vi "Lockin.DAQ.Trigger.vi"(8 "error in (no error)":errorcluster, 11 "Lockin.DAQ":refnum<class "Lockin.DAQ.lvclass">) -> (0 "error out":errorcluster, 3 "Lockin.DAQ":refnum<class "Lockin.DAQ.lvclass">)   [LabVIEW 2016, in "Lockin.DAQ.lvclass"]
uses:
  Lockin.DAQ.lvclass
  Typedefs/DAQType-enum.ctl
  Lockin.DAQ.lvclass/Lockin.DAQ.ctl
  <vilib>/DAQmx/configure/trigger.llb/DAQmx Start Trigger (Digital Edge).vi
  <userlib>/_OpenG.lib/array/array.llb/Remove Duplicates from 1D Array (Variant)__ogtk.vi
  <resource>/objmgr/daqmx.rc
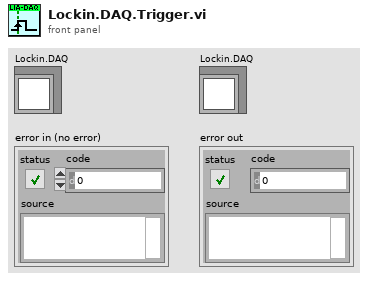
[diagram p1: front panel]
types:
  T1 = typedef "Lockin.DAQ.lvclass/DAQType-enum.ctl" = enum16{"None", "USB 4431", "PXI 446x"}
  T2 = cluster{"DAQ Type":T1, "Master Tasks":refnum<k21>[], "RefClk.Src":tag, "SyncPulse.Src":tag, "Trigger.Src":tag, "SyncPulse.SyncTime":dbl}
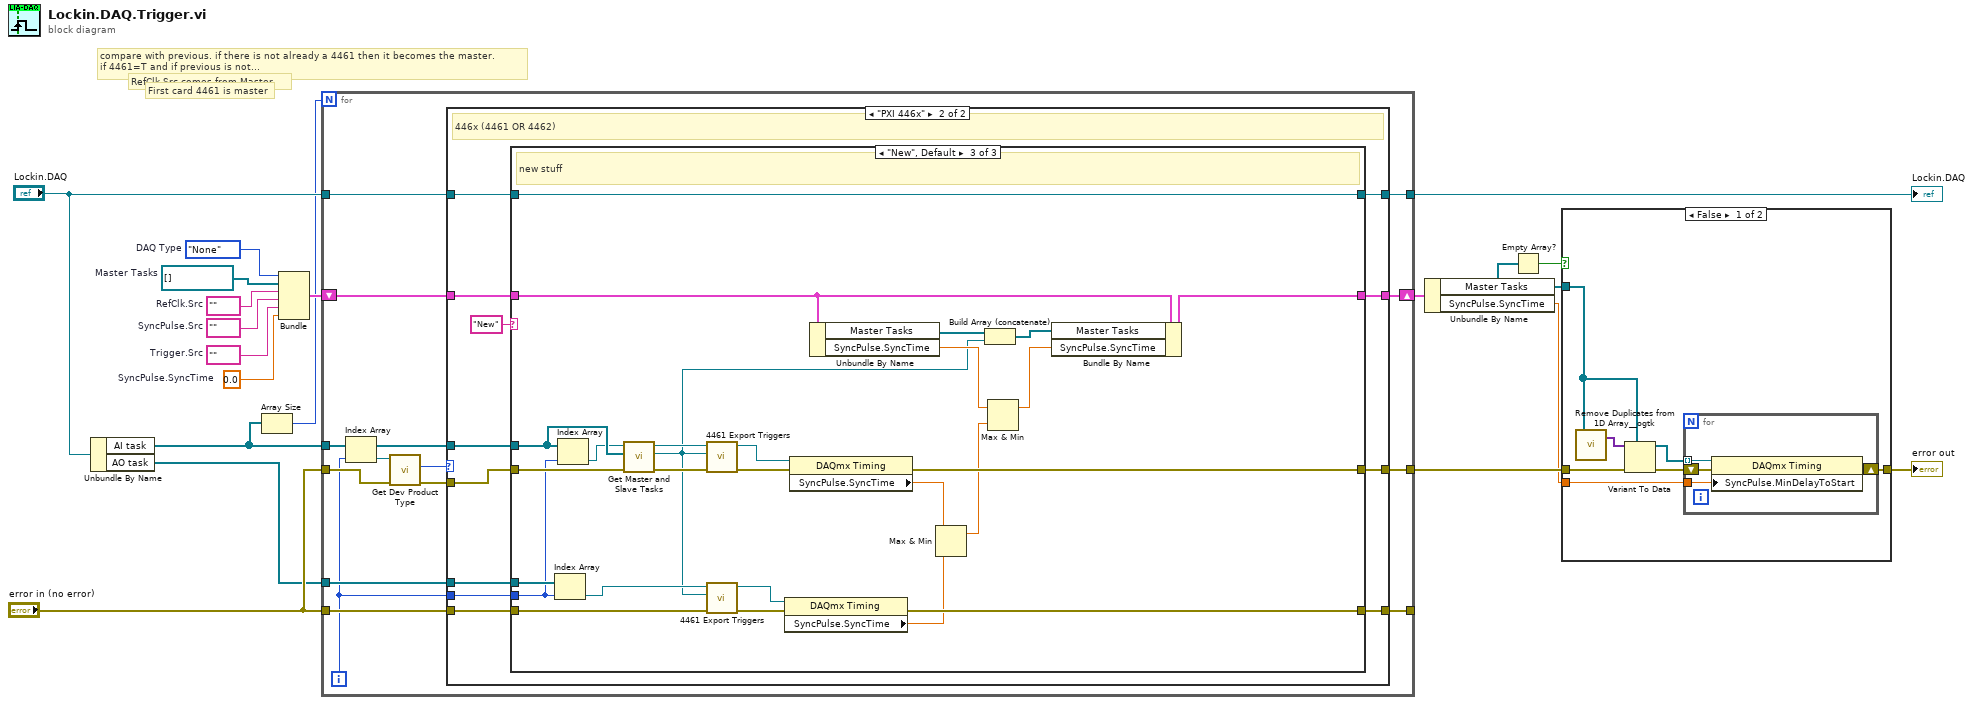
[diagram p0: block diagram]
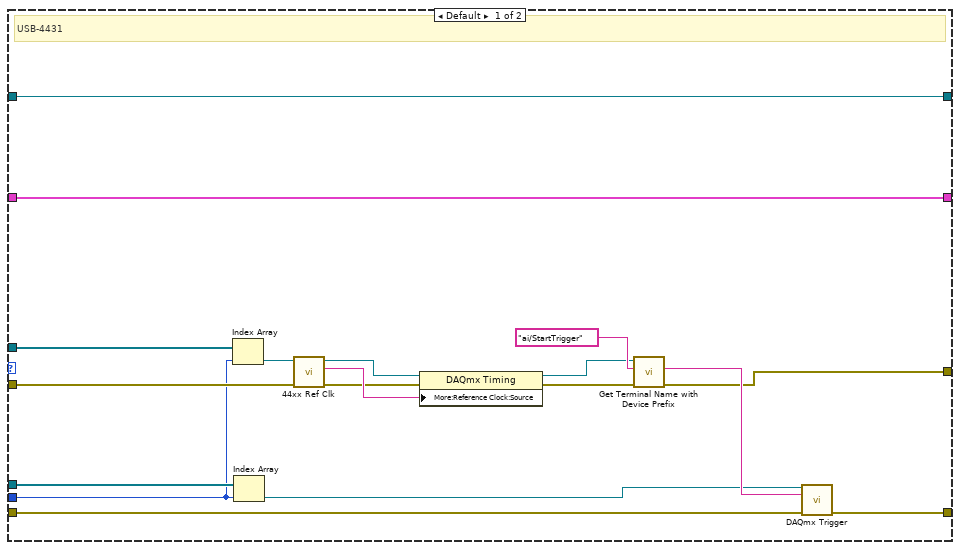
[diagram p2: hidden frame]
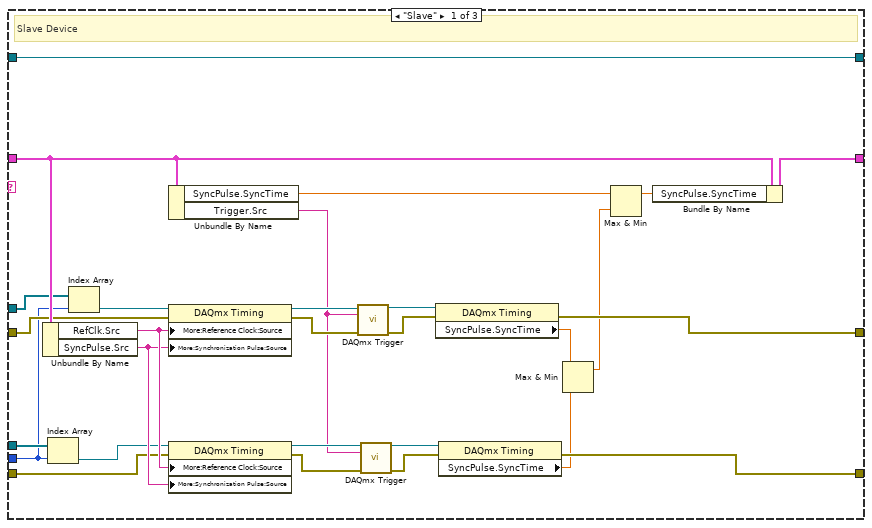
[diagram p3: hidden frame]
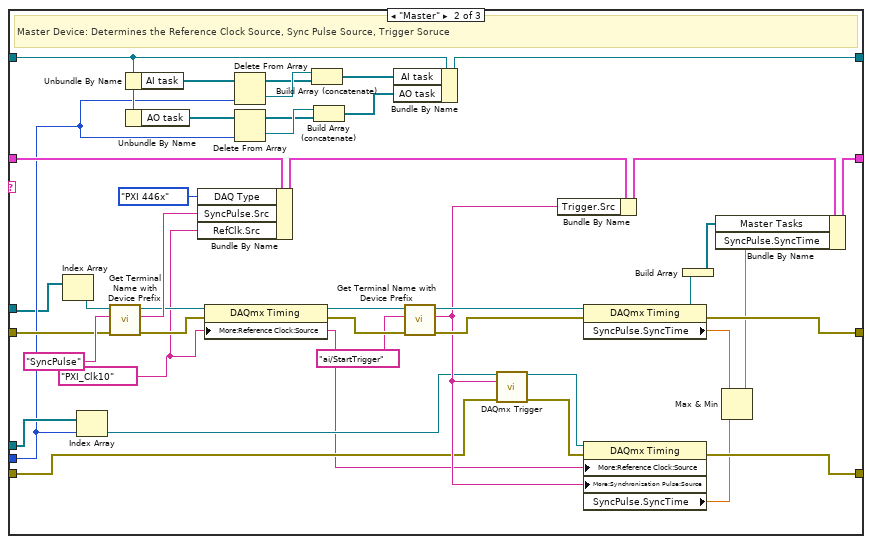
[diagram p4: hidden frame]
diagram:
  w1 = refnum<k21>[] []  # Master Tasks
  w13 = 0.0  # SyncPulse.SyncTime
  w12 = tag ""  # Trigger.Src
  w11 = tag ""  # SyncPulse.Src
  w5 = tag ""  # RefClk.Src
  w4 = DAQType-enum."None"  # DAQ Type
  # "RefClk.Src comes from Master"
  # "compare with previous. if there is not already a 4461 then it becomes the master. \nif 4461=T and if previous is not..."
  # "First card 4461 is master"
  n1 = Unbundle By Name("Lockin.DAQ") -> ("AI task"=w2:refnum<k21>[], "AO task"=w6:refnum<k21>[])
  n2 = Array Size(array=w2) -> (size(s)=w3:i32)
  n3 = Bundle("DAQ Type"=w4, "Master Tasks"=w1, "RefClk.Src"=w5, "SyncPulse.Src"=w11, "Trigger.Src"=w12, "SyncPulse.SyncTime"=w13) -> (w10:T2)  [unwired: 1 in]
  n4 = for {
    N: w3 -> [_]
    tunnel: w2 -> [w21]
    tunnel: "error in (no error)" -> [w33]
    shift-right: [w31] -> w14
    shift-left: w10 -> [w32]
    tunnel: [w30] -> w18
    tunnel: "Lockin.DAQ" -> [w29]
    tunnel: [w28] -> w8
    tunnel: [w27] -> _
    tunnel: "error in (no error)" -> [w26]
    tunnel: w6 -> [w23]
    i -> [w22]
    n5 = Index Array(array=w21, index=w22) -> (element=w24:refnum<k21>)
    n6 = call "Get Dev Product Type.vi"("error in (no error)"=w33, "Refnum in"=w24) -> ("error out"=w20:errorcluster, "DAQ Type"=w25:T1)  [unwired: 6 in, 2 out]
    n7 = case shown="\"PXI 446x\"" w25 {
      tunnel: w32 -> [w51 w63]
      tunnel: [w51 w62] -> w31
      tunnel: w20 -> [w38 w61]
      tunnel: [w42 w60] -> w30
      tunnel: w29 -> [w50 w59]
      tunnel: [w50 w58] -> w28
      tunnel: [w43 w55] -> w27
      tunnel: w26 -> [w44 w57]
      tunnel: w23 -> [w46 w56]
      tunnel: w22 -> [w35 w54]
      tunnel: w21 -> [w36 w53]
      frame Default {
        # "USB-4431"
        n8 = Index Array(array=w36, index=w35) -> (element=w34:refnum<k21>)
        n9 = Index Array(array=w46, index=w35) -> (element=w41:refnum<k21>)
        n10 = call "44xx Ref Clk.vi"("error in (no error)"=w38, "Refnum in"=w34) -> ("error out"=w37:errorcluster, "RefClk.Src"=w40:tag, "Refnum out"=w39:refnum<k21>)  [unwired: 7 in]
        n11 = property class="DAQmx Timing"(reference=w39, error in=w37, "More:Reference Clock:Source"=w40) -> (reference out=w48:refnum<k21>, error out=w47:errorcluster)
        n12 = call "Get Terminal Name with Device Prefix.vi"("error in (no error)"=w47, "Local Terminal Name"="ai/StartTrigger", "task/channels in"=w48) -> ("error out"=w42:errorcluster, "Terminal Name with Device Prefix"=w45:tag)  [unwired: 6 in, 1 out]
        n13 = call-poly <vilib>:"DAQmx Trigger.vi"("task/channels in"=w41, "source"=w45, "error in"=w44) -> ("error out"=w43:errorcluster)  [unwired: 11 in, 1 out]
      }
      frame "PXI 446x" {
        # "446x (4461 OR 4462)"
        n14 = case shown="\"New\", Default" "New" {
          tunnel: w63 -> [w89 w133 w140]
          tunnel: [w88 w122 w141] -> w62
          tunnel: w61 -> [w76 w130 w152]
          tunnel: [w86 w121 w158] -> w60
          tunnel: w59 -> [w85 w111 w154]
          tunnel: [w85 w113 w154] -> w58
          tunnel: w57 -> [w69 w102 w150]
          tunnel: w56 -> [w68 w99 w153]
          tunnel: [w75 w112 w157] -> w55
          tunnel: w54 -> [w65 w98 w149]
          tunnel: w53 -> [w66 w95 w143]
          frame "Slave" {
            # "Slave Device"
            n15 = Unbundle By Name(w89) -> ("RefClk.Src"=w84:tag, "SyncPulse.Src"=w83:tag)
            n16 = Index Array(array=w68, index=w65) -> (element=w67:refnum<k21>)
            n17 = Index Array(array=w66, index=w65) -> (element=w64:refnum<k21>)
            n18 = Unbundle By Name(w89) -> ("SyncPulse.SyncTime"=w72:dbl, "Trigger.Src"=w79:tag)
            n19 = property class="DAQmx Timing"(reference=w64, error in=w76, "More:Reference Clock:Source"=w84, "More:Synchronization Pulse:Source"=w83) -> (reference out=w91:refnum<k21>, error out=w80:errorcluster)
            n20 = property class="DAQmx Timing"(reference=w67, error in=w69, "More:Reference Clock:Source"=w84, "More:Synchronization Pulse:Source"=w83) -> (reference out=w81:refnum<k21>, error out=w78:errorcluster)
            n21 = call-poly <vilib>:"DAQmx Trigger.vi"("task/channels in"=w91, "source"=w79, "error in"=w80) -> ("task out"=w90:refnum<k21>, "error out"=w87:errorcluster)  [unwired: 11 in]
            n22 = call-poly <vilib>:"DAQmx Trigger.vi"("task/channels in"=w81, "source"=w79, "error in"=w78) -> ("task out"=w82:refnum<k21>, "error out"=w77:errorcluster)  [unwired: 11 in]
            n23 = property class="DAQmx Timing"(reference=w90, error in=w87) -> (error out=w86:errorcluster, "SyncPulse.SyncTime"=w70:dbl)  [unwired: 1 out]
            n24 = property class="DAQmx Timing"(reference=w82, error in=w77) -> (error out=w75:errorcluster, "SyncPulse.SyncTime"=w74:dbl)  [unwired: 1 out]
            n25 = Max & Min(x=w70, y=w74) -> (max(x,y)=w73:dbl)  [unwired: 1 out]
            n26 = Max & Min(x=w72, y=w73) -> (max(x,y)=w71:dbl)  [unwired: 1 out]
            n27 = Bundle By Name(cluster=w89, "SyncPulse.SyncTime"=w71) -> (w88:T2)
          }
          frame "Master" {
            w94 = tag "PXI_Clk10" ("RefClk.Src")
            # "Master Device: Determines the Reference Clock Source, Sync Pulse Source, Trigger Soruce"
            n28 = Index Array(array=w95) -> (element=w96:refnum<k21>)  [unwired: 1 in]
            n29 = Index Array(array=w99, index=w98) -> (element=w97:refnum<k21>)
            n30 = call "Get Terminal Name with Device Prefix.vi"("error in (no error)"=w130, "Local Terminal Name"="SyncPulse", "task/channels in"=w96) -> ("error out"=w129:errorcluster, "Terminal Name with Device Prefix"=w131:tag, "task out"=w119:refnum<k21>)  [unwired: 6 in]
            n31 = Unbundle By Name(w111) -> ("AI task"=w117:refnum<k21>[])
            n32 = Unbundle By Name(w111) -> ("AO task"=w110:refnum<k21>[])
            n33 = Bundle By Name(cluster=w133, "DAQ Type"=DAQType-enum."PXI 446x", "SyncPulse.Src"=w131, "RefClk.Src"=w94) -> (w125:T2)
            n34 = property class="DAQmx Timing"(reference=w119, error in=w129, "More:Reference Clock:Source"=w94) -> (reference out=w126:refnum<k21>, error out=w128:errorcluster)
            n35 = Delete From Array(array=w117, index=w98) -> (deleted portion=w116:refnum<k21>, array with subset deleted=w115:refnum<k21>[])  [unwired: 1 in]
            n36 = Delete From Array(array=w110, index=w98) -> (deleted portion=w109:refnum<k21>, array with subset deleted=w108:refnum<k21>[])  [unwired: 1 in]
            n37 = Build Array (concatenate)(w116, w115) -> (w114:refnum<k21>[])
            n38 = Build Array (concatenate)(w109, w108) -> (w107:refnum<k21>[])
            n39 = Bundle By Name(cluster=w111, "AI task"=w114, "AO task"=w107) -> (w113:refnum<class "Lockin.DAQ.lvclass">)
            n40 = call "Get Terminal Name with Device Prefix.vi"("error in (no error)"=w128, "Local Terminal Name"="ai/StartTrigger", "task/channels in"=w126) -> ("error out"=w123:errorcluster, "Terminal Name with Device Prefix"=w103:tag, "task out"=w124:refnum<k21>)  [unwired: 6 in]
            n41 = call-poly <vilib>:"DAQmx Trigger.vi"("task/channels in"=w97, "source"=w103, "error in"=w102) -> ("task out"=w100:refnum<k21>, "error out"=w101:errorcluster)  [unwired: 11 in]
            n42 = Bundle By Name(cluster=w125, "Trigger.Src"=w103) -> (w120:T2)
            n43 = property class="DAQmx Timing"(reference=w124, error in=w123) -> (reference out=w118:refnum<k21>, error out=w121:errorcluster, "SyncPulse.SyncTime"=w106:dbl)
            n44 = property class="DAQmx Timing"(reference=w100, error in=w101, "More:Reference Clock:Source"=w94, "More:Synchronization Pulse:Source"=w103) -> (error out=w112:errorcluster, "SyncPulse.SyncTime"=w105:dbl)  [unwired: 1 out]
            n45 = Build Array(w118) -> (w92:refnum<k21>[])
            n46 = Max & Min(x=w106, y=w105) -> (max(x,y)=w104:dbl)  [unwired: 1 out]
            n47 = Bundle By Name(cluster=w120, "Master Tasks"=w92, "SyncPulse.SyncTime"=w104) -> (w122:T2)
          }
          frame "New", Default {
            # "new stuff"
            n48 = Index Array(array=w153, index=w149) -> (element=w147:refnum<k21>)
            n49 = Index Array(array=w143, index=w149) -> (element=w142:refnum<k21>)
            n50 = call "Get Master and Slave Tasks.vi"("error in (no error)"=w152, "AI tasks in"=w143, "AI task"=w142) -> ("error out"=w151:errorcluster, "master task"=w134:refnum<k21>, "AI task out"=w148:refnum<k21>)  [unwired: 6 in]
            n51 = call "4461 Export Triggers.vi"("error in (no error)"=w151, "master task in"=w134, "task in"=w148) -> ("error out"=w159:errorcluster, "task out"=w146:refnum<k21>)  [unwired: 7 in]
            n52 = call "4461 Export Triggers.vi"("error in (no error)"=w150, "master task in"=w134, "task in"=w147) -> ("error out"=w144:errorcluster, "task out"=w145:refnum<k21>)  [unwired: 7 in]
            n53 = property class="DAQmx Timing"(reference=w145, error in=w144) -> (error out=w157:errorcluster, "SyncPulse.SyncTime"=w155:dbl)  [unwired: 1 out]
            n54 = property class="DAQmx Timing"(reference=w146, error in=w159) -> (error out=w158:errorcluster, "SyncPulse.SyncTime"=w156:dbl)  [unwired: 1 out]
            n55 = Unbundle By Name(w140) -> ("Master Tasks"=w136:refnum<k21>[], "SyncPulse.SyncTime"=w138:dbl)
            n56 = Max & Min(x=w156, y=w155) -> (max(x,y)=w139:dbl)  [unwired: 1 out]
            n57 = Build Array (concatenate)(w136, w134) -> (w135:refnum<k21>[])
            n58 = Max & Min(x=w138, y=w139) -> (max(x,y)=w137:dbl)  [unwired: 1 out]
            n59 = Bundle By Name(cluster=w140, "Master Tasks"=w135, "SyncPulse.SyncTime"=w137) -> (w141:T2)
          }
        }
      }
    }
  }
  "Lockin.DAQ" <- w8
  n60 = Unbundle By Name(w14) -> ("Master Tasks"=w16:refnum<k21>[], "SyncPulse.SyncTime"=w17:dbl)
  n61 = Empty Array?(array=w16) -> (empty?=w15:bool)
  n62 = case shown="False" w15 {
    tunnel: w16 -> [w163 _]
    tunnel: w17 -> [w166 _]
    tunnel: w18 -> [w161 w171]
    tunnel: [w165 w171] -> w19
    frame False {
      n63 = call-poly <userlib>:"Remove Duplicates from 1D Array__ogtk.vi"("Input Array"=w163) -> ("Output Array"=w164:variant[])  [unwired: 1 out]
      n64 = Variant To Data(error in=w161, type=w163, Variant=w164) -> (data=w162:refnum<k21>[], error out=w160:errorcluster)
      n65 = for {
        tunnel: w166 -> [w170]
        shift-right: [w168] -> w165
        shift-left: w160 -> [w169]
        tunnel: w162 -> [w167] mode=indexing
        n66 = property class="DAQmx Timing"(reference=w167, error in=w169, "SyncPulse.MinDelayToStart"=w170) -> (error out=w168:errorcluster)  [unwired: 1 out]
      }
    }
    frame True {
      # "If master task=empty, then no master devices were ever found (ie, all 4431s)"
    }
  }
  "error out" <- w19
